vi "ControlHeadingWithRudder.vi"(0 "Desired Heading":dbl, 1 "Robot Heading":dbl) -> (7 "Suggested Rudder Setpoint":T2 min=-1.0 max=1.0)   [LabVIEW 2013]
doc: "Takes in an angle to check, and returns a goodness value related to how close said angle is to the angle between the robot and the waypoint.\n\n**I find the above statement very unclear. What this vi should do now (perhaps this wasn't the original point, I can't tell) is take in the angle of the boat relative to the target, and use the rudder to point the boat at the target. This is done by putting a control loop around the boat-to-waypoint angle and making it go to zero. The control loop should be adjusted so that you get a more extreme reaction from the rudder at lower speeds. At a very low speed cutoff perhaps the rudder should just be set to 0, to save battery from the rudder twitching back and forth.**\n\nModified by Eric Schneider, Jan. 2014"
uses:
  Data/TypeDefs/UTM Location.ctl
  Data/TypeDefs/Rudder Set Suggestions.ctl
  <vilib>/addons/control/pid/NI_PID_autopid.lvlib
panel:
  in  "Start the autotuning?":bool
  out "tuning completed?":bool
  out "PID gains out":T1={"proportional gain (Kc)"=1.0, "integral time (Ti, min)"=0.01, "derivative time (Td, min)"=0.0} {"derivative time (Td, min)" format="%.3f"; "integral time (Ti, min)" format="%.3f"; "proportional gain (Kc)" format="%.3f"}
  in  "Robot Location":T3 {"North" format="%#_10f"; "East" format="%#_8f"}
  in  "Waypoint":T3 {"North" format="%#_10f"; "East" format="%#_8f"}
  # "PID autotuning details"
  # "TODO: Pass this 'start\nautotuning' switch up\ninto the OCU"
  # "Do we need these? Depends on how desired\nheading is calculated, I think"
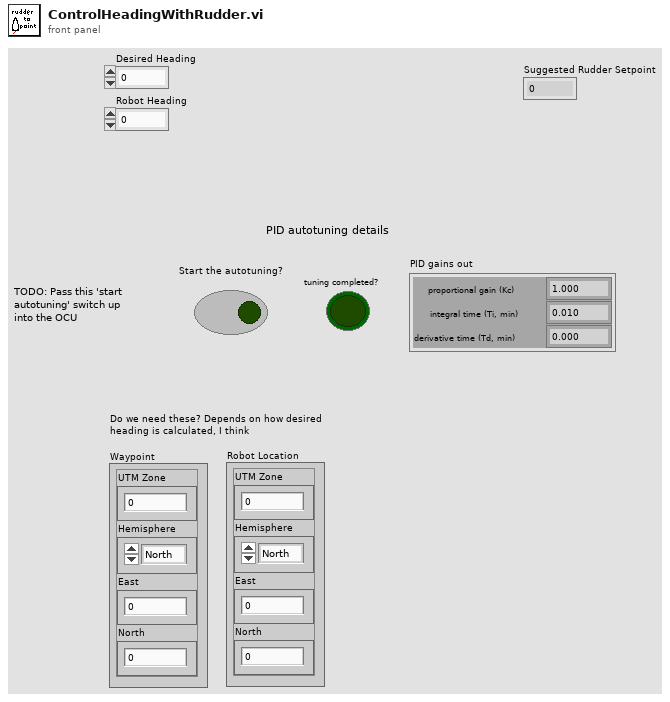
[diagram p1: front panel]
types:
  T1 = cluster{"proportional gain (Kc)":dbl, "integral time (Ti, min)":dbl, "derivative time (Td, min)":dbl}
  T2 = typedef "Rudder Set Suggestions.ctl" = dbl
  T3 = typedef "UTM Location.ctl" = cluster{"UTM Zone":dbl, "Hemisphere":enum16{"North", "South"}, "East":dbl, "North":dbl}
  T4 = cluster{"controller type":u16, "relay cycles":i32, "relay amplitude":dbl, "control specification":u16, "PV noise level":dbl}
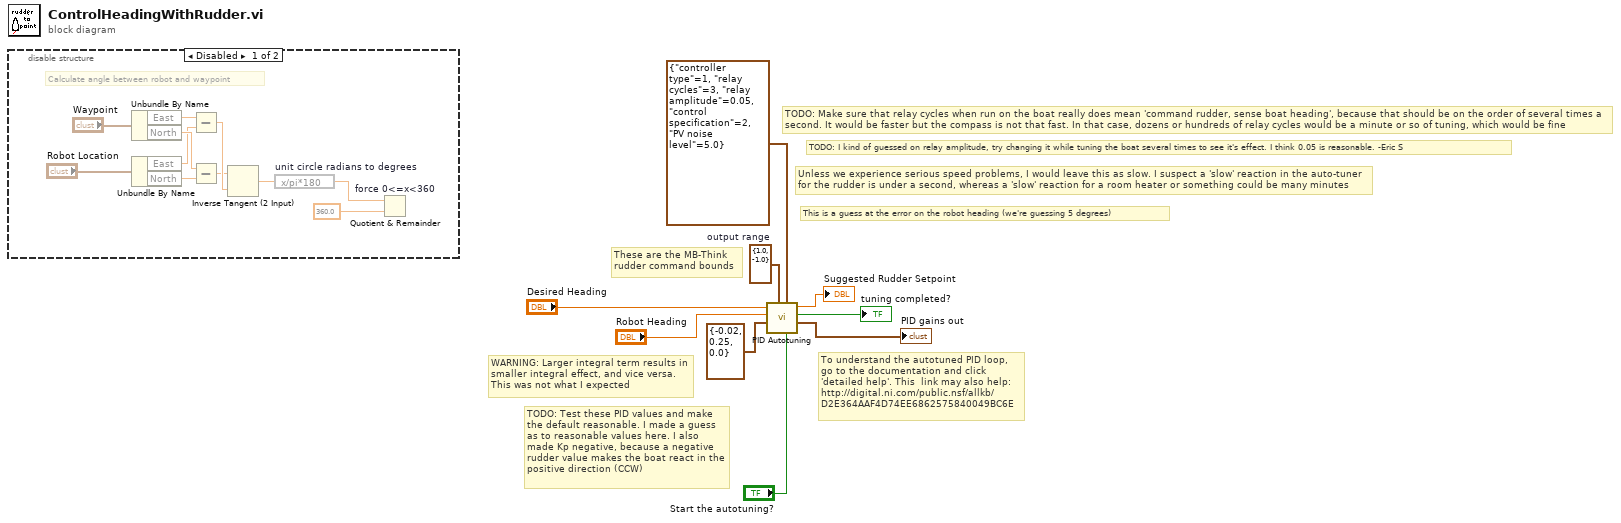
[diagram p0: block diagram]
diagram:
  w6 = cluster{"output high":dbl, "output low":dbl} {"output high"=1.0, "output low"=-1.0}  # output range
  # "WARNING: Larger integral term results in smaller integral effect, and vice versa. This was not what I expected"
  # "These are the MB-Think rudder command bounds"
  # "TODO: Test these PID values and make the default reasonable. I made a guess as to reasonable values here. I also made Kp negative, because a negative rudder value makes the boat react in the positive direction (CCW)"
  # "This is a guess at the error on the robot heading (we're guessing 5 degrees)"
  # "Unless we experience serious speed problems, I would leave this as slow. I suspect a 'slow' reaction in the auto-tuner for the rudder is under a second, whereas a 'slow' reaction for a room heater or something could be many minutes"
  # "TODO: I kind of guessed on relay amplitude, try changing it while tuning the boat several times to see it's effect. I think 0.05 is reasonable. -Eric S"
  # "TODO: Make sure that relay cycles when run on the boat really does mean 'command rudder, sense boat heading', because that should be on the order of several times a second. It would be faster but the compass is not that fast. In that case, dozens or hundreds of relay cycles would be a minute or so of tuning, which would be fine"
  # "To understand the autotuned PID loop, go to the documentation and click 'detailed help'. This  link may also help: http://digital.ni.com/public.nsf/allkb/D2E364AAF4D74EE6862575840049BC6E"
  n1 = disable-structure shown="Disabled" {
    frame Disabled {
      # "Calculate angle between robot and waypoint"
      n2 = Unbundle By Name("Waypoint") -> ("East"=w15:dbl, "North"=w17:dbl)
      n3 = Unbundle By Name("Robot Location") -> ("East"=w16:dbl, "North"=w18:dbl)
      n4 = Subtract(x=w15, y=w16) -> (x-y=w20:dbl)
      n5 = Subtract(x=w17, y=w18) -> (x-y=w19:dbl)
      n6 = Inverse Tangent (2 Input) ("use inverse tangent\nto get heading")(1:w20, 2:w19) -> (0:w11:dbl)
      n7 = expression code="x/pi*180" "unit circle radians to degrees"(w11) -> (w10:dbl)
      n8 = Quotient & Remainder "force 0<=x<360"(x=w10, y=360.0) -> ()  [unwired: 2 out]
    }
    frame Enabled {
    }
  }
  n9 = call <vilib>:"PID Autotuning.vi"("autotune? (F)"="Start the autotuning?", "autotuning parameters"=T4 {"controller type"=1, "relay cycles"=3, "relay amplitude"=0.05, "control specification"=2, "PV noise level"=5.0}, "output range"=w6, "PID gains"=T1 {"proportional gain (Kc)"=-0.02, "integral time (Ti, min)"=0.25, "derivative time (Td, min)"=0.0}, "process variable"="Robot Heading", "setpoint"="Desired Heading") -> ("PID gains out"=→"PID gains out":T1, "tuning completed?"=→"tuning completed?":bool, "output"=→"Suggested Rudder Setpoint":dbl)  [unwired: 2 in, 1 out]
